vi "SpinBridge_SubVI.vi"(10 "Motor Spin in":i32, 11 "BrickReference in":T1) -> (3 "BrickReference out":T1)   [LabVIEW 2016]
uses:
  <vilib>/NXT/Subs/LVHSConnector.ctl
  <vilib>/NXT/LegoClasses/BrickReference/BrickReference.lvclass
  <vilib>/NXT/Block Support/NXT_OutputPort.ctl
  <vilib>/NXT/NXTIO Xnodes/NXTIONodeSubVIs/NXTMotorRunDistance.vi
  <vilib>/NXT/Dual Mode Library/Waits/Wait_Num.vi
  <vilib>/NXT/NXTIO Xnodes/AddressXNode/NXTIOAddress.xnode
  <vilib>/NXT/NXTIO Xnodes/NXTIOXNode/NXTIO.xnode
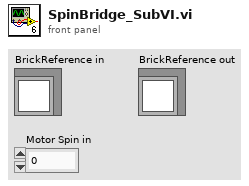
[diagram p1: front panel]
types:
  T1 = typedef "LVHSConnector.ctl" = refnum<class "BrickReference.lvclass">
  T2 = typedef "NXT_OutputPort.ctl" = u8
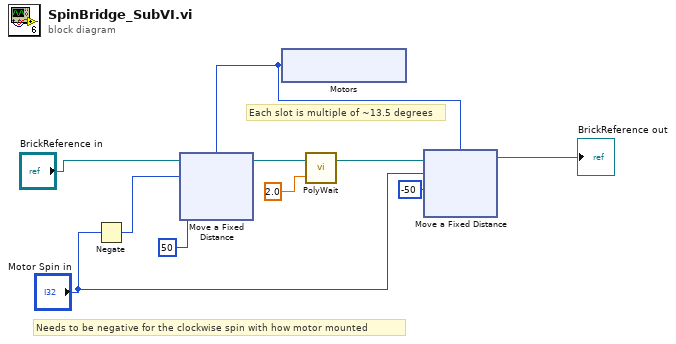
[diagram p0: block diagram]
diagram:
  # "Needs to be negative for the clockwise spin with how motor mounted"
  # "Each slot is multiple of ~13.5 degrees"
  n1 = Negate(x="Motor Spin in") -> (-x=w6:i32)
  n2 = xnode "Motors"() -> ("Motor"=w5:T2)
  n3 = xnode "Move a Fixed Distance"("Speed 1"=i8 50, "Distance 1"=w6, "Motors"=w5, "NXT/EV3"="BrickReference in") -> ("NXT/EV3"=w8:T1)
  n4 = call-poly <vilib>:"PolyWait.vi"("Time (1 sec)"=sgl 2.0, "NXT/EV3"=w8) -> ("NXT/EV3"=w9:T1)  [unwired: 2 in]
  n5 = xnode "Move a Fixed Distance"("Speed 1"=i8 -50, "Distance 1"="Motor Spin in", "Motors"=w5, "NXT/EV3"=w9) -> ("NXT/EV3"=→"BrickReference out":T1)
